vi "Abort or Close Running VIs.vi"() -> ()   [LabVIEW 2025]
doc: "Utility to close a modal VI when it has been brought to the foreground and reserved to run. This locks up LabVIEW so this VI will present a list of VIs to optionally close.\nScott Hannahs, National High Magnetic Field Lab\nJanuary 2005\n<sth@magnet.fsu.edu>"
panel:
  in  "Write-in VI's to abort":string[](array[string])
  out "Slide 2":i32(slide) scale=-1.0..1.0
  in  "VIs to Abort":i32[](listbox)
  in  "OK Button":bool
  in  "VIs to close":i32[](listbox)
  out "Slide":i32(slide)
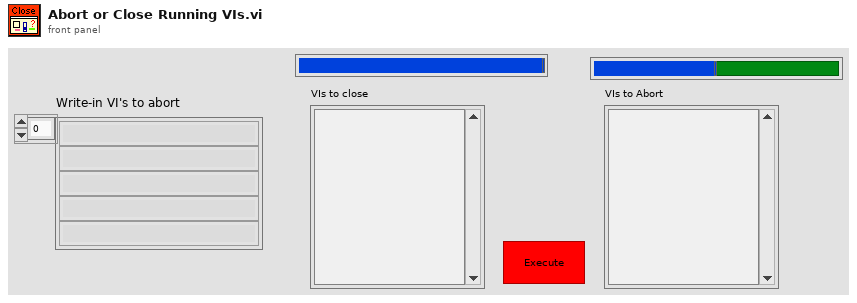
[diagram p1: front panel]
types:
  T1 = enum32{"Bad", "Idle", "Run top level", "Running"}
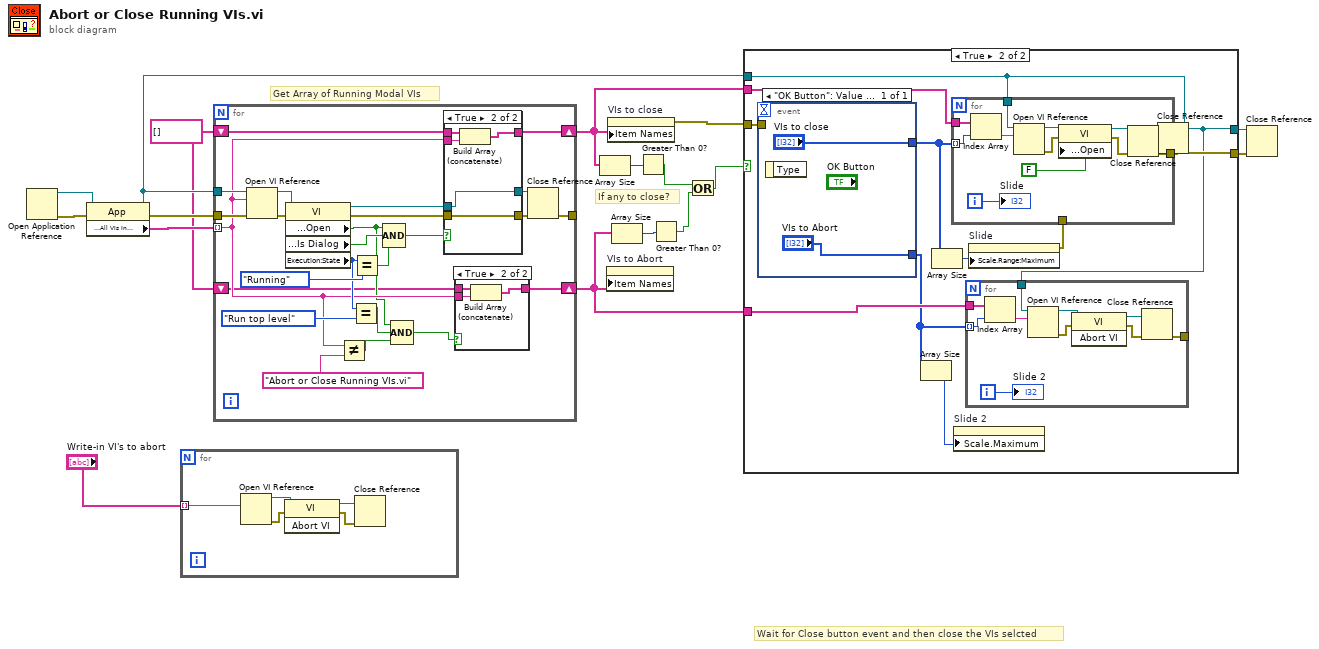
[diagram p0: block diagram]
diagram:
  w8 = string[] []
  # "If any to close?"
  # "Wait for Close button event and then close the VIs selcted"
  # "Get Array of Running Modal VIs"
  n1 = Open Application Reference() -> (0:w17:errorcluster, 3:w16:refnum<vi>)  [unwired: 4 in]
  n2 = property class="App"(reference=w16, error in=w17) -> (reference out=w11:refnum<vi>, error out=w15:errorcluster, "Application:All VIs In Memory"=w14:string[])
  n3 = for {
    tunnel: "Write-in VI's to abort" -> [w18] mode=indexing
    n4 = Open VI Reference(vi path=w18) -> (vi reference=w22:refnum<vi>, error out=w21:errorcluster)  [unwired: 5 in]
    n5 = invoke class="VI" method="Abort VI"(reference=w22, error in=w21) -> (reference out=w20:refnum<vi>, error out=w19:errorcluster)  [unwired: 1 in, 1 out]
    n6 = Close Reference(reference=w20, error in (no error)=w19) -> ()  [unwired: 1 out]
  }
  n7 = for {
    tunnel: w15 -> [w47]
    tunnel: w14 -> [w29] mode=indexing
    tunnel: w11 -> [w36]
    tunnel: [w39] -> _
    shift-right: [w35] -> w12
    shift-left: w8 -> [w32]
    shift-right: [w30] -> w2
    shift-left: w8 -> [w23]
    n8 = Open VI Reference(application reference (local)=w36, vi path=w29, error in (no error)=w47) -> (vi reference=w45:refnum<vi>, error out=w46:errorcluster)  [unwired: 3 in]
    n9 = property class="VI"(reference=w45, error in=w46) -> (reference out=w42:refnum<vi>, error out=w31:errorcluster, "Front Panel Window:Open"=w27:bool, "Front Panel Window:Is Dialog"=w44:bool, "Execution:State"=w33:T1)
    n10 = Not Equal?(x=w29, y="Abort or Close Running VIs.vi") -> (x != y?=w25:bool)
    n11 = Equal?(x=w33, y=T1."Run top level") -> (x = y?=w26:bool)
    n12 = Equal?(x=w33, y=T1."Running") -> (x = y?=w37:bool)
    n13 = Compound Arithmetic op=AND(w27, w44, w37) -> (w43:bool)
    n14 = Compound Arithmetic op=AND(w27, w26, w25) -> (w24:bool)
    n15 = case shown="True" w43 {
      tunnel: w31 -> [w53 w57]
      tunnel: w42 -> [w54 w55]
      tunnel: [w53 w57] -> w41
      tunnel: [w54 w55] -> w40
      tunnel: w32 -> [w52 w59]
      tunnel: w29 -> [_ w58]
      tunnel: [w52 w56] -> w35
      frame False {
      }
      frame True {
        n16 = Build Array (concatenate)(w59, w58) -> (w56:string[])
      }
    }
    n17 = case shown="True" w24 {
      tunnel: w23 -> [w48 w51]
      tunnel: w29 -> [_ w50]
      tunnel: [w48 w49] -> w30
      frame False {
      }
      frame True {
        n18 = Build Array (concatenate)(w51, w50) -> (w49:string[])
      }
    }
    n19 = Close Reference(reference=w40, error in (no error)=w41) -> (error out=w39:errorcluster)
  }
  n20 = Array Size(array=w12) -> (size(s)=w7:i32)
  n21 = property on="VIs to Abort" class="LstBox (strict)"("Item Names"=w2) -> ()  [unwired: 2 in, 2 out]
  n22 = property on="VIs to close" class="LstBox (strict)"("Item Names"=w12) -> (error out=w13:errorcluster)  [unwired: 2 in, 1 out]
  n23 = Array Size(array=w2) -> (size(s)=w6:i32)
  n24 = Greater Than 0?(x=w7) -> (x > 0?=w5:bool)
  n25 = Greater Than 0?(x=w6) -> (x > 0?=w4:bool)
  n26 = Or(x=w5, y=w4) -> (x .or. y?=w3:bool)
  n27 = case shown="True" w3 {
    tunnel: w13 -> [w61 w70]
    tunnel: [w61 w67] -> w9
    tunnel: w12 -> [_ w66]
    tunnel: w11 -> [w60 w64]
    tunnel: [w60 w64] -> w10
    tunnel: w2 -> [_ w65]
    frame False {
    }
    frame True {
      n28 = event shown="[0] \"OK Button\": Value Change" {
        selector: _ -> [_]
        dyn-events: _ -> [_]
        timeout: _ -> [_]
        tunnel: w70 -> [_]
        tunnel: ["VIs to close"] -> w69
        tunnel: ["VIs to Abort"] -> w63
        event "OK Button": Value Change {
          n29 = event-data() -> ()  [unwired: 1 in, 1 out]
        }
      }
      n30 = Array Size(array=w63) -> (size(s)=w62:i32)
      n31 = Array Size(array=w69) -> (size(s)=w71:i32)
      n32 = property on="Slide 2" class="Slide (strict)"("Scale.Maximum"=w62) -> ()  [unwired: 2 in, 2 out]
      n33 = for {
        tunnel: w63 -> [w78] mode=indexing
        tunnel: w65 -> [w79]
        tunnel: w64 -> [w73]
        tunnel: [w72] -> _
        i -> [w81]
        n34 = Index Array(array=w79, index=w78) -> (element=w80:string)
        n35 = Open VI Reference(application reference (local)=w73, vi path=w80) -> (vi reference=w77:refnum<vi>, error out=w76:errorcluster)  [unwired: 4 in]
        n36 = invoke class="VI" method="Abort VI"(reference=w77, error in=w76) -> (reference out=w75:refnum<vi>, error out=w74:errorcluster)  [unwired: 1 in, 1 out]
        n37 = Close Reference(reference=w75, error in (no error)=w74) -> (error out=w72:errorcluster)
        "Slide 2" <- w81
      }
      n38 = property on="Slide" class="Slide (strict)"("Scale.Range:Maximum"=w71) -> (error out=w68:errorcluster)  [unwired: 2 in, 1 out]
      n39 = for {
        tunnel: w69 -> [w89] mode=indexing
        tunnel: w68 -> [_]
        tunnel: w66 -> [w90]
        tunnel: w64 -> [w83]
        tunnel: [w82] -> w67
        i -> [w92]
        n40 = Index Array(array=w90, index=w89) -> (element=w91:string)
        n41 = Open VI Reference(application reference (local)=w83, vi path=w91) -> (vi reference=w88:refnum<vi>, error out=w87:errorcluster)  [unwired: 4 in]
        n42 = property class="VI"(reference=w88, error in=w87, "Front Panel Window:Open"=FALSE) -> (reference out=w85:refnum<vi>, error out=w84:errorcluster)
        n43 = Close Reference(reference=w85, error in (no error)=w84) -> (error out=w82:errorcluster)
        "Slide" <- w92
      }
    }
  }
  n44 = Close Reference(reference=w10, error in (no error)=w9) -> ()  [unwired: 1 out]
  n45 = Close Reference(reference=w10, error in (no error)=w9) -> ()  [unwired: 1 out]
